vi "FTW-Container-Element-SetVariant.vi"(0 "FTW-Container In":refnum<class "FTW-Container.lvclass">, 7 "Variant":variant, 11 "error in":errorcluster) -> (4 "FTW-Container Out":refnum<class "FTW-Container.lvclass">, 8 "Replaced":bool, 15 "error out":errorcluster)   [LabVIEW 2015, in "FTW-Container.lvclass"]
uses:
  FTW-Container.lvclass
  FTW-Container.lvclass/FTW-Container.ctl
  <vilib>/Utility/Data Type/NI_Data Type.lvlib
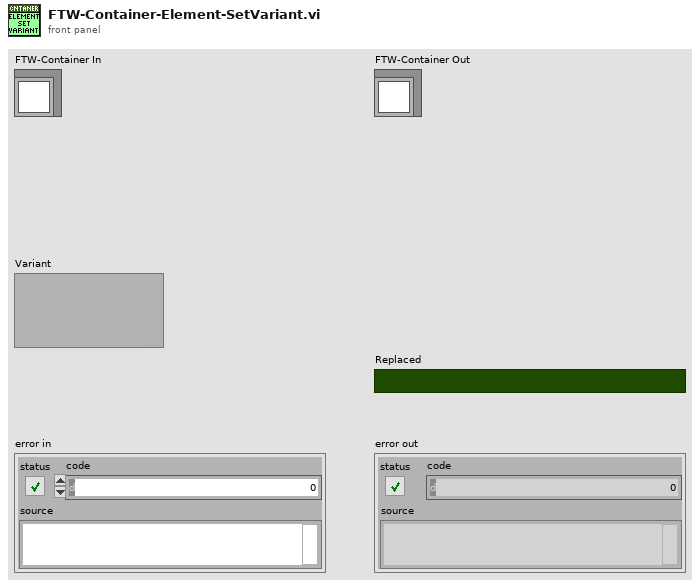
[diagram p1: front panel]
types:
  T1 = typedef "NI_Data Type.lvlib/Data Type.ctl" = enum8{"Invalid Type", "Void", "I8", "I16", "I32", "I64", "U8", "U16", "U32", "U64", "Single Float", "Double Float", "Extended Float", "Single Complex", "Double Complex", "Extended Complex", "Enum U8", "Enum U16", "Enum U32", "Enum U64", "Single Float With Unit", "Double Float With Unit", "Extended Float With Unit", "Single Complex with Unit", "Double Complex with Unit", "Extended Complex with Unit", "Boolean", "String", "Path", "Picture", "Tag", "Array", "Cluster", "Variant", "LV Variant", "Waveform", "Timestamp", "Digital Waveform", "Digital Data", "ExpressData", "Refnum", "External Data", "VI", "Poly VI", "LabVIEW Class Instance", "Fixed Point"}
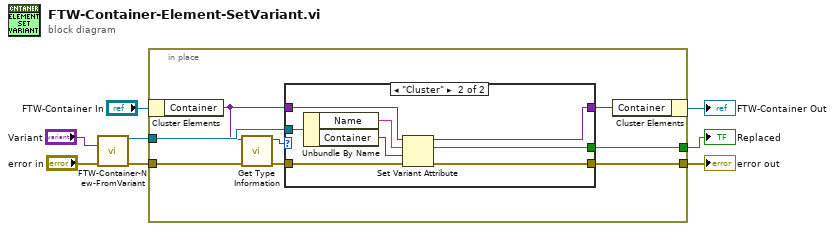
[diagram p0: block diagram]
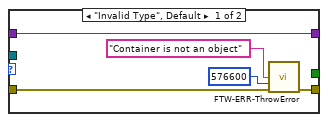
[diagram p2: hidden frame]
diagram:
  n1 = call "FTW-Container-New-FromVariant.vi"("Variant"="Variant", "error in"="error in") -> ("FTW-Container"=w1:refnum<class "FTW-Container.lvclass">, "error out"=w3:errorcluster)  [unwired: 12 in]
  n2 = in-place {
    in-place-border: [w15] -> w6
    in-place-border: w3 -> [w16]
    in-place-border: w1 -> [w11]
    in-place-border: [w9] -> w4
    n3 = in-place-cluster #1("FTW-Container In") -> ("Container"=w10:variant)
    n4 = call <vilib>:"Get Type Information.vi"("error in (no error)"=w16, "Variant"=w10) -> ("error out"=w13:errorcluster, "Type"=w12:T1)  [unwired: 5 in, 3 out]
    n5 = case shown="\"Cluster\"" w12 {
      tunnel: w13 -> [w19 w29]
      tunnel: [w18 w28] -> w15
      tunnel: w10 -> [w17 w27]
      tunnel: [w17 w25] -> w14
      tunnel: w11 -> [_ w26]
      tunnel: [_ w24] -> w9
      frame "Invalid Type", Default {
        n6 = call "FTW-ERR-ThrowError.vi"("Error Message"="Container is not an object", "Error Code"=576600, "error in"=w19) -> ("error out"=w18:errorcluster)  [unwired: 12 in]
      }
      frame "Cluster" {
        n7 = Unbundle By Name(w26) -> ("Name"=w22:string, "Container"=w23:variant)
        n8 = Set Variant Attribute(Variant=w27, name=w22, value=w23, error in=w29) -> (Variant out=w25:variant, replaced=w24:bool, error out=w28:errorcluster)
      }
    }
    n9 = in-place-cluster #1("Container"=w14) -> (→"FTW-Container Out":refnum<class "FTW-Container.lvclass">)
  }
  "error out" <- w6
  "Replaced" <- w4
